vi "Row_Set Cell Values (numeric).vi"(7 "format (%.3f)":string="%.3f", 8 "error in (no error)":errorcluster, 9 "text data (row)":dbl[](array[numeric]), 10 "Row":refnum<k24>, 11 "ooWriter in":refnum<class "ooCalc.lvclass">) -> (0 "error out":errorcluster, 3 "ooWriter out":refnum<class "ooCalc.lvclass">)   [LabVIEW 2009, in "ooCalc.lvclass"]
uses:
  ooCalc.lvclass
  C:/Projets/LAVAG/OpenOfficeRGT/AODL/DLLs/AODL.dll
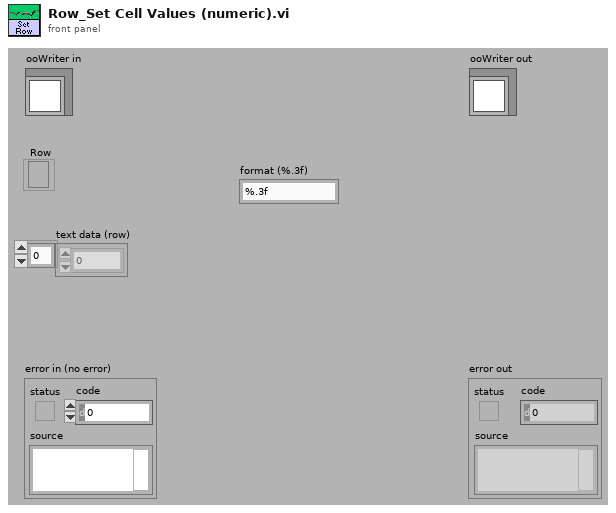
[diagram p1: front panel]
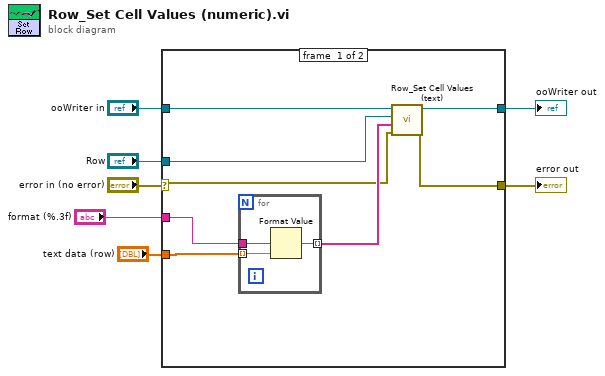
[diagram p0: block diagram]
diagram:
  n1 = case shown="No Error" "error in (no error)" {
    selector: "error in (no error)" -> [w9 w20]
    tunnel: [w8 w20] -> w6
    tunnel: [w14 w19] -> w4
    tunnel: "ooWriter in" -> [w15 w19]
    tunnel: "text data (row)" -> [w12 _]
    tunnel: "Row" -> [w13 _]
    tunnel: "format (%.3f)" -> [w11 _]
    frame #0 {
      n2 = for {
        tunnel: w12 -> [w18] mode=indexing
        tunnel: w11 -> [w17]
        tunnel: [w16] -> w10 mode=indexing
        n3 = Format Value(format string=w17, value (0)=w18) -> (output string=w16:string)  [unwired: 1 in]
      }
      n4 = call-dynamic "Row_Set Cell Values (text).vi"("error in (no error)"=w9, "text data (row)"=w10, "Row"=w13, "ooWriter in"=w15) -> ("error out"=w8:errorcluster, "ooWriter out"=w14:refnum<class "ooCalc.lvclass">)  [unwired: 6 in]
    }
    frame #1 {
    }
  }
  "error out" <- w6
  "ooWriter out" <- w4
